vi "Is Line Detector Available.vi"(8 "Error In":errorcluster) -> (0 "Error Out":errorcluster, 2 "Execution:State":T1(ring), 3 "Good":bool)   [LabVIEW 2016]
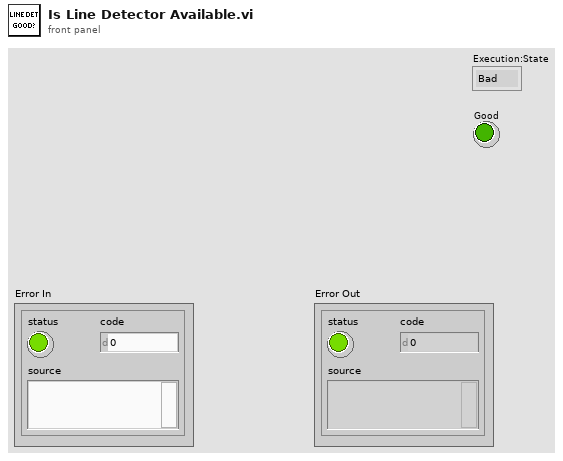
[diagram p1: front panel]
types:
  T1 = enum32{"Bad", "Idle", "Run top level", "Running"}
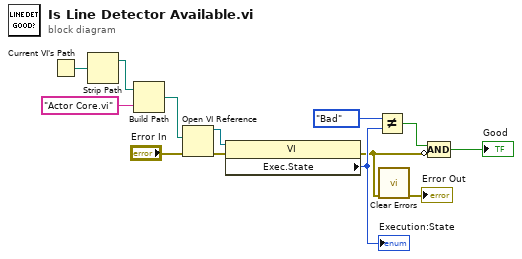
[diagram p0: block diagram]
diagram:
  n1 = Current VI's Path() -> (path=w12:path)
  n2 = Strip Path(path=w12) -> (stripped path=w11:path)  [unwired: 1 out]
  n3 = Build Path(base path=w11, name or relative path="Actor Core.vi") -> (appended path=w8:path)
  n4 = Open VI Reference(vi path=w8, error in (no error)="Error In") -> (vi reference=w9:refnum<vi>, error out=w10:errorcluster)  [unwired: 4 in]
  n5 = property class="VI"(reference=w9, error in=w10) -> (error out=w2:errorcluster, "Exec.State"=w7:T1)  [unwired: 1 out]
  "Execution:State" <- w7
  n6 = Not Equal?(x=T1."Bad" ("Execution:State"), y=w7) -> (x != y?=w4:bool)
  n7 = call <vilib>:"Clear Errors.vi"("error in (no error)"=w2) -> ("error out"=→"Error Out":errorcluster)  [unwired: 5 in, 1 out]
  n8 = Compound Arithmetic op=AND(w4, invert w2) -> (→"Good":bool)
